vi "get_middle_element_of_array.vi"(11 "array in":dbl[](array[numeric])) -> (0 "even(t)/odd(f) array length":bool, 1 "middle element of array (I32)":i32, 2 "middle element of array (dbl)":dbl, 3 "array out":dbl[](array[numeric]), 4 "middle element of array (string)":string)   [LabVIEW 2018]
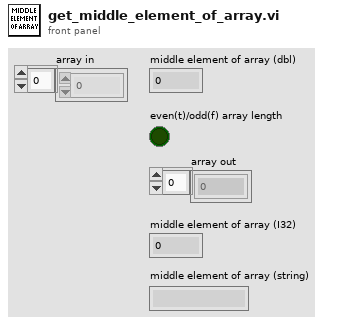
[diagram p1: front panel]
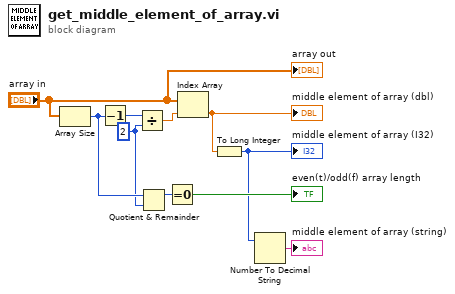
[diagram p0: block diagram]
diagram:
  w7 = 2 ("y")
  n1 = Array Size(array="array in") -> (size(s)=w8:i32)
  n2 = Decrement(x=w8) -> (x-1=w9:i32)
  n3 = Divide(x=w9, y=w7) -> (x/y=w10:dbl)
  n4 = Quotient & Remainder(x=w8, y=w7) -> (x-y*floor(x/y)=w6:i32)  [unwired: 1 out]
  n5 = Equal To 0?(x=w6) -> (x = 0?=→"even(t)/odd(f) array length":bool)
  n6 = Index Array(array="array in", index=w10) -> (element=w3:dbl)
  "middle element of array (dbl)" <- w3
  n7 = To Long Integer(number=w3) -> (32bit integer=w1:i32)
  "middle element of array (I32)" <- w1
  n8 = Number To Decimal String(number=w1) -> (decimal integer string=→"middle element of array (string)":string)  [unwired: 1 in]
  "array out" <- "array in"
